vi "VISA IDN SIM900 Fix.vi"(6 "Manufacturer in":string="Stanford_Research_Systems", 7 "Revision in":string="ver3.6", 8 "error in (no error)":errorcluster {"code" format="%.0x"}, 9 "Info in":string="s/n130040", 10 "Model in":string="SIM900", 11 "VISA Resource Name":refnum<visa-resource-name>="GPIB0::3::INSTR") -> (0 "error out":errorcluster {"code" format="%.0x"}, 2 "Devices":T1[](array[typedef]) {"Status" format="%.0x"}, 3 "dup VISA Session":refnum<visa-resource-name>)   [LabVIEW 2020]
uses:
  New NML Data Acq/Sub Controls/Instrument IDN.ctl
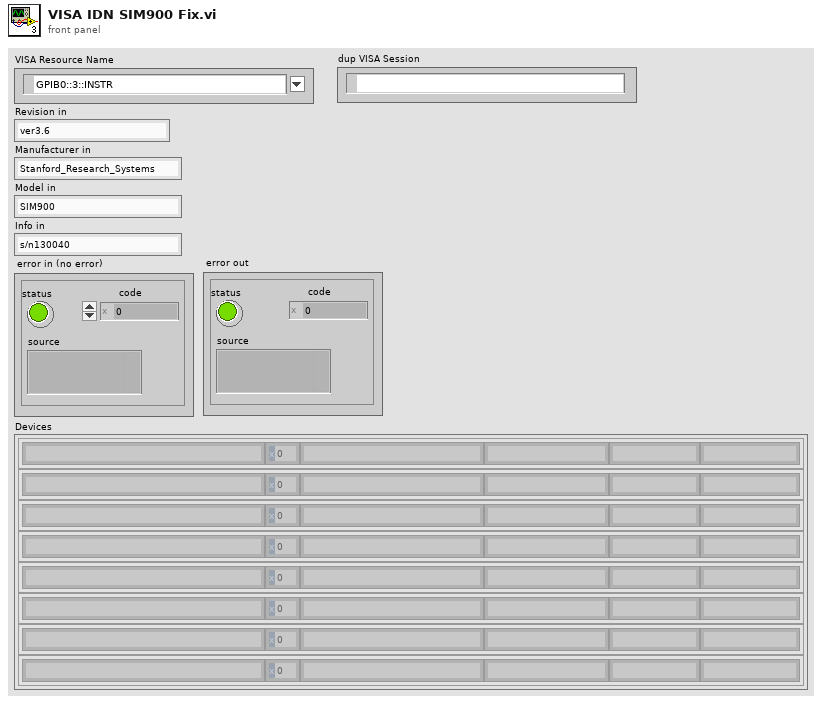
[diagram p1: front panel]
types:
  T1 = typedef "Instrument IDN.ctl" = cluster{"VISA Address":string, "Status":u16, "Manufacturer":string, "Model":string, "Info":string, "Info 2":string, "Misc Data":variant}
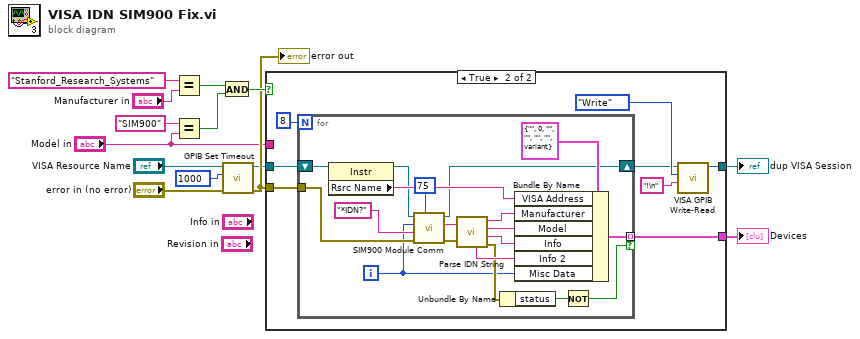
[diagram p0: block diagram]
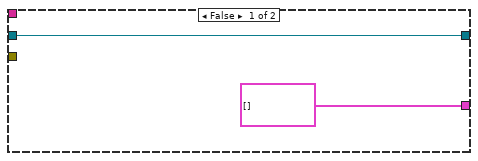
[diagram p2: hidden frame]
diagram:
  n1 = Equal?(x="Stanford_Research_Systems" ("y"), y="Manufacturer in") -> (x = y?=w12:bool)
  n2 = Equal?(x="SIM900" ("y"), y="Model in") -> (x = y?=w6:bool)
  n3 = And(x=w12, y=w6) -> (x .and. y?=w14:bool)
  n4 = call "GPIB Set Timeout.vi"("Error In"="error in (no error)", "Timeout"=u32 1000, "VISA resource name"="VISA Resource Name") -> ("Error Out"=w9:errorcluster, "dup VISA resource name"=w2:refnum<visa-resource-name>)  [unwired: 2 in, 1 out]
  "error out" <- w9
  n5 = case shown="True" w14 {
    tunnel: "Model in" -> [_ _]
    tunnel: w9 -> [_ w18]
    tunnel: [T1[] [] w17] -> w1
    tunnel: w2 -> [w15 w19]
    tunnel: [w15 w21] -> w8
    frame False {
    }
    frame True {
      n6 = for {
        N: 8 -> [_]
        tunnel: [w38] -> w17 mode=indexing if=w34
        shift-right: [w30] -> w20
        shift-left: w19 -> [w26]
        tunnel: w18 -> [w32]
        i -> [w28]
        n7 = property class="Instr"(reference=w26) -> (reference out=w25:refnum<visa-resource-name>, "Rsrc Name"=w37:string)  [unwired: 1 in, 1 out]
        n8 = call "SIM900 Module Comm.vi"("Wait (ms)"=u32 75, "Error In"=w32, "Query"="*IDN?" ("write buffer (\"\")"), "Slot"=w28, "VISA Resource Name"=w25) -> ("Error Out"=w29:errorcluster, "Response"=w31:string, "dup VISA Session"=w30:refnum<visa-resource-name>)  [unwired: 4 in]
        n9 = call "Parse IDN String.vi"("error in (no error)"=w29, "IDN String"=w31) -> ("error out"=w36:errorcluster, "Info"=w42:string, "Model"=w41:string, "Manufacturer"=w39:string, "Revision"=w40:string)
        n10 = Unbundle By Name(w36) -> ("status"=w35:bool)
        n11 = Bundle By Name(cluster=T1 {"VISA Address"="", "Status"=0, "Manufacturer"="", "Model"="", "Info"="", "Info 2"="", "Misc Data"=variant} ("Instrument List"), "VISA Address"=w37, "Manufacturer"=w39, "Model"=w41, "Info"=w42, "Info 2"=w40, "Misc Data"=w28) -> (w38:T1)
        n12 = Not(x=w35) -> (.not. x?=w34:bool)
      }
      n13 = call "VISA GPIB Write-Read.vi"("Command"="!\n", "Action"=enum16{"Write", "Read", "Write & Read"}."Write", "VISA resource name"=w20) -> ("dup VISA Session"=w21:refnum<visa-resource-name>)  [unwired: 5 in, 3 out]
    }
  }
  "Devices" <- w1
  "dup VISA Session" <- w8
